vi "WireErrorControlsToConnectorPane.vi"(6 "Error terminals":T1, 8 "error in (no error)":errorcluster, 11 "VI":refnum<vi>) -> (0 "error out":errorcluster, 3 "VI (dup)":refnum<vi>)   [LabVIEW 2017, in "ErrorStructureDrawer.lvlib"]
doc: "Wires the error control and indicator into the connector pane"
uses:
  ErrorStructureDrawer.lvlib
  Controls/ErrorTerminals.ctl
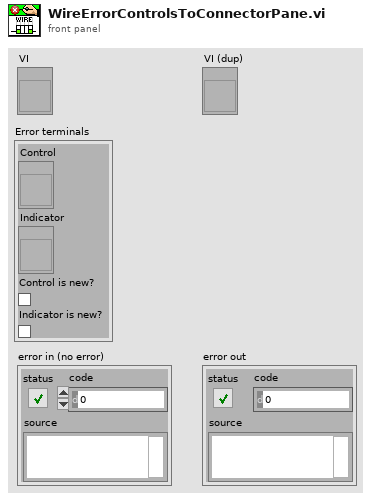
[diagram p1: front panel]
types:
  T1 = typedef "ErrorStructureDrawer.lvlib/ErrorTerminals.ctl" = cluster{"Control":refnum<vi>, "Indicator":refnum<vi>, "Control is new?":bool, "Indicator is new?":bool}
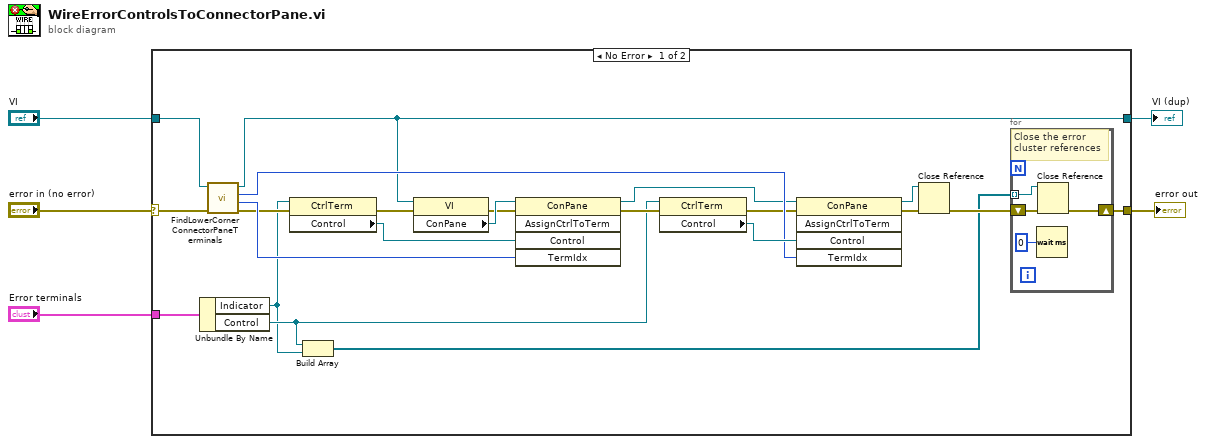
[diagram p0: block diagram]
diagram:
  n1 = case shown="No Error" "error in (no error)" {
    selector: "error in (no error)" -> [w9 w33]
    tunnel: "Error terminals" -> [w27 _]
    tunnel: [w26 w33] -> w4
    tunnel: [w17 w32] -> w3
    tunnel: "VI" -> [w15 w32]
    frame No Error {
      n2 = Unbundle By Name(w27) -> ("Indicator"=w7:refnum<vi>, "Control"=w8:refnum<vi>)
      n3 = call "FindLowerCornerConnectorPaneTerminals.vi"("error in (no error)"=w9, "VI reference"=w15) -> ("error out"=w13:errorcluster, "Bottom right index"=w22:u32, "Bottom left index"=w21:u32, "VI reference (dup)"=w17:refnum<vi>)  [unwired: 6 in]
      n4 = property class="CtrlTerm"(reference=w7, error in=w13) -> (error out=w14:errorcluster, "Control"=w24:refnum<vi>)  [unwired: 1 out]
      n5 = Build Array(w8, w7) -> (w6:refnum<vi>[])
      n6 = property class="VI"(reference=w17, error in=w14) -> (error out=w16:errorcluster, "ConPane"=w18:refnum<vi>)  [unwired: 1 out]
      n7 = invoke class="ConPane" method="AssignCtrlToTerm"(reference=w18, error in=w16, "Control"=w24, "TermIdx"=w22) -> (reference out=w10:refnum<vi>, error out=w12:errorcluster)  [unwired: 1 in, 3 out]
      n8 = property class="CtrlTerm"(reference=w8, error in=w12) -> (error out=w11:errorcluster, "Control"=w23:refnum<vi>)  [unwired: 1 out]
      n9 = invoke class="ConPane" method="AssignCtrlToTerm"(reference=w10, error in=w11, "Control"=w23, "TermIdx"=w21) -> (reference out=w20:refnum<vi>, error out=w19:errorcluster)  [unwired: 1 in, 3 out]
      n10 = Close Reference(reference=w20, error in (no error)=w19) -> (error out=w25:errorcluster)
      n11 = for {
        tunnel: w6 -> [w31] mode=indexing
        shift-right: [w29] -> w26
        shift-left: w25 -> [w30]
        # "Close the error cluster references"
        n12 = Wait (ms)(milliseconds to wait=u32 0) -> ()  [unwired: 1 out]
        n13 = Close Reference(reference=w31, error in (no error)=w30) -> (error out=w29:errorcluster)
      }
    }
    frame Error {
    }
  }
  "error out" <- w4
  "VI (dup)" <- w3
